vi "FX1s.vi"() -> ()   [LabVIEW 2017]
panel:
  out "Open":i32
  in  "lpsData 2":i16
  in  "lpsData":i16
  in  "停止":bool
  in  "ActUtlType":refnum<k7>(container)
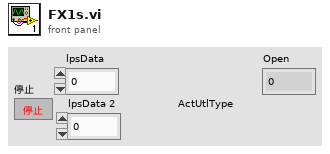
[diagram p1: front panel]
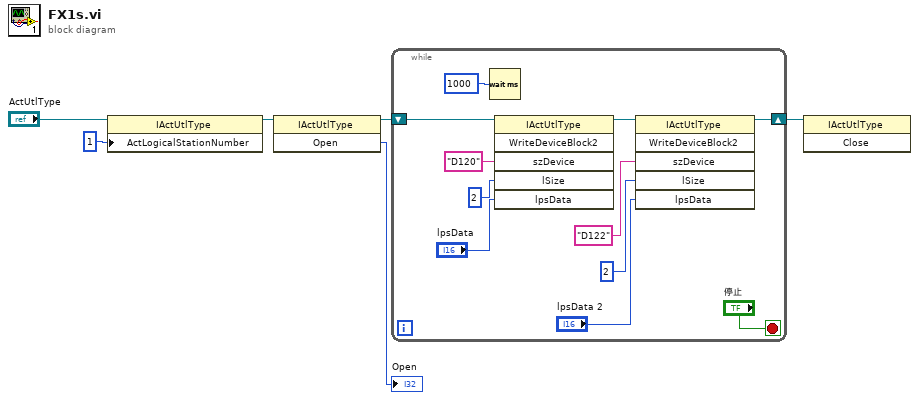
[diagram p0: block diagram]
diagram:
  n1 = property class="IActUtlType"(reference="ActUtlType", "ActLogicalStationNumber"=1) -> (reference out=w4:refnum<k7>)  [unwired: 1 in, 1 out]
  n2 = invoke class="IActUtlType" method="Open"(reference=w4) -> (reference out=w3:refnum<k7>, "Open"=→"Open":i32)  [unwired: 2 in, 1 out]
  n3 = while {
    shift-right: [w9] -> w2
    shift-left: w3 -> [w17]
    stop <- "停止" stop-if-true
    n4 = Wait (ms)(milliseconds to wait=u32 1000 ("等待时间（毫秒）")) -> ()  [unwired: 1 out]
    n5 = invoke class="IActUtlType" method="WriteDeviceBlock2"(reference=w17, "szDevice"="D120" ("szDeviceList"), "lSize"=2, "lpsData"="lpsData") -> (reference out=w10:refnum<k7>)  [unwired: 2 in, 5 out]
    n6 = invoke class="IActUtlType" method="WriteDeviceBlock2"(reference=w10, "szDevice"="D122" ("szDeviceList"), "lSize"=2, "lpsData"="lpsData 2") -> (reference out=w9:refnum<k7>)  [unwired: 2 in, 5 out]
  }
  n7 = invoke class="IActUtlType" method="Close"(reference=w2) -> ()  [unwired: 2 in, 3 out]
